vi "BRig_dataBlock_nTrial_biasing.vi"() -> (2 "output_nTrial_biasing":i32)   [LabVIEW 2014]
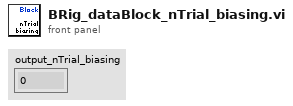
[diagram p1: front panel]
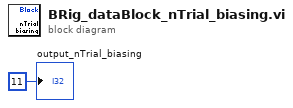
[diagram p0: block diagram]
diagram:
  "output_nTrial_biasing" <- 11 ("output_iBlock")
